vi "radar_plot_tracks.vi"(3 "error in":errorcluster, 5 "Radar Sample":T1) -> (0 "error out":errorcluster)   [LabVIEW 2019, in "Lib_Simx.lvlib"]
doc: "Tool to plot distance away of the radar on the x and y axis."
uses:
  Lib_Simx.lvlib
  controls/radarSample.ctl
  controls/RadarTrack.ctl
  <vilib>/Utility/miscctls.llb/LVAnnotationListTypeDef.ctl
panel:
  in  "Show Track ID":bool
  out "Plot Tracks":cluster{"X1":dbl[], "Y1":dbl[]}[](graph)
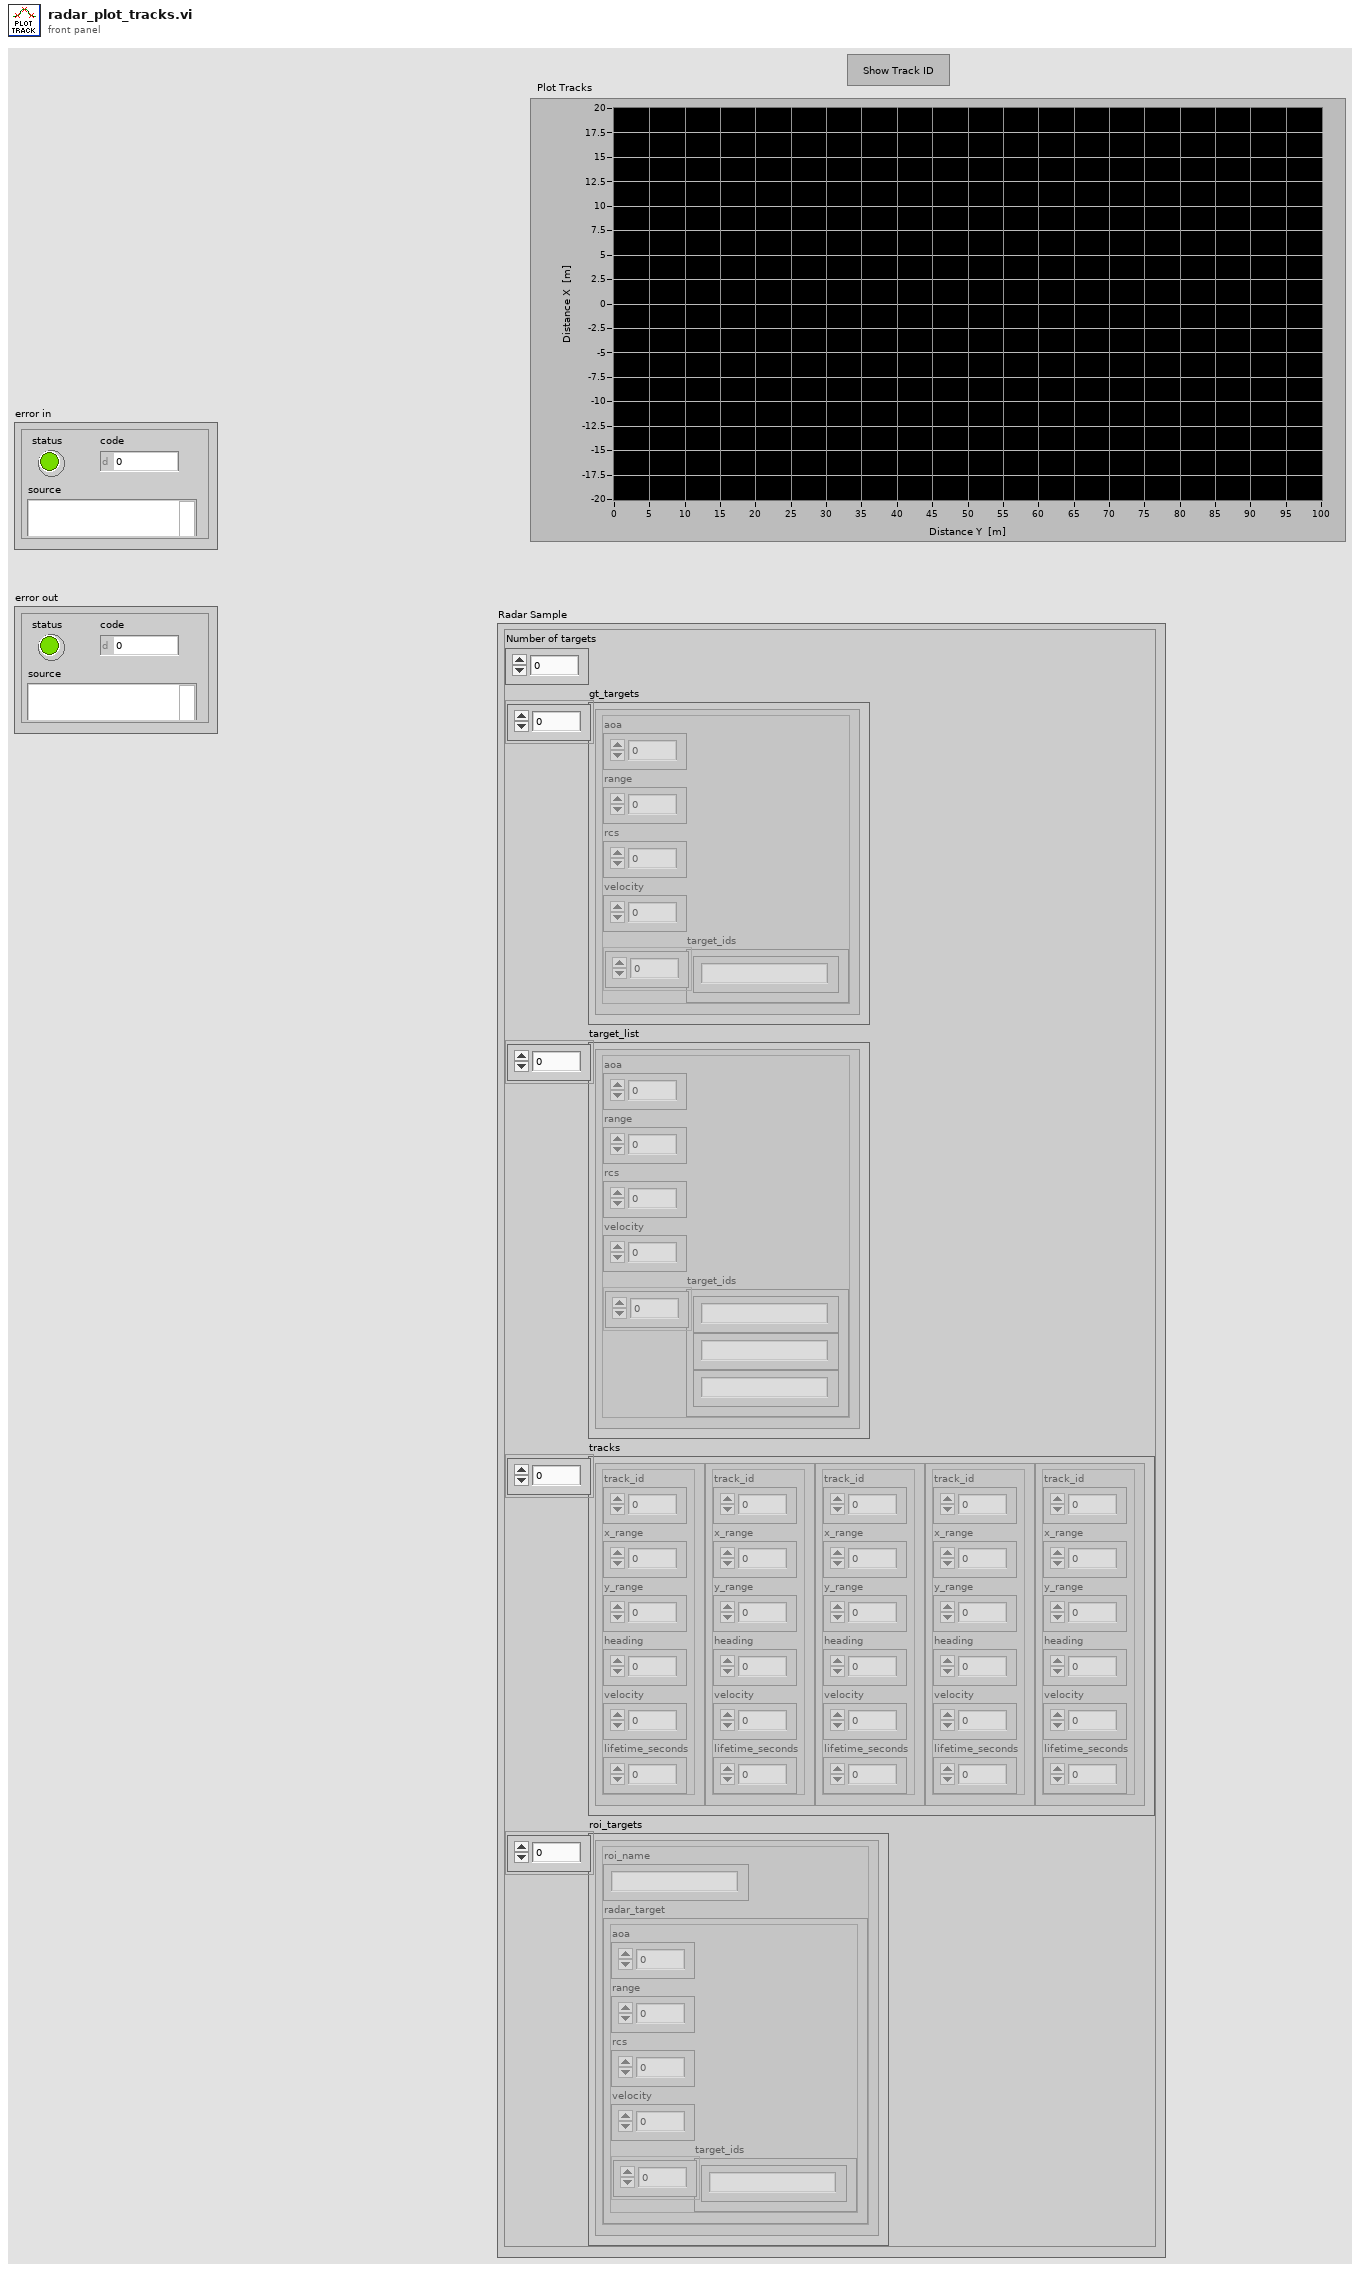
[diagram p1: front panel]
types:
  T1 = typedef "Lib_Simx.lvlib/radarSample.ctl" = cluster{"Number of targets":i32, "gt_targets":cluster{"aoa":sgl, "range":sgl, "rcs":sgl, "velocity":sgl, "target_ids":string[]}[], "target_list":cluster{"aoa":sgl, "range":sgl, "rcs":sgl, "velocity":sgl, "target_ids":string[]}[], "tracks":T2[], "roi_targets":cluster{"roi_name":string, "radar_target":cluster{"aoa":sgl, "range":sgl, "rcs":sgl, "velocity":sgl, "target_ids":string[]}}[]}
  T2 = typedef "Lib_Simx.lvlib/RadarTrack.ctl" = cluster{"track_id":u64, "x_range":sgl, "y_range":sgl, "heading":sgl, "velocity":sgl, "lifetime_seconds":sgl}
  T3 = cluster{"Name":string, "Color":u32, "Style":u8, "Point Style":u8, "Name Visible":bool, "Allow Drag":bool, "Annotation Mode":u32, "Plot":i32, "Index":i32, "Position":cluster{"X":dbl, "Y":dbl}, "X Scale":u32, "Y Scale":u32, "Show Arrow":bool, "Lock Name":bool, "Plot Area":i32, "Label Offset":cluster{"X":dbl, "Y":dbl}}
  T4 = typedef "LVAnnotationListTypeDef.ctl" = cluster{"Name":string, "Color":u32, "Style":u8, "Point Style":u8, "Name Visible":bool, "Allow Drag":bool, "Annotation Mode":u32, "Plot":i32, "Index":i32, "Position":cluster{"X":dbl, "Y":dbl}, "X Scale":u32, "Y Scale":u32, "Show Arrow":bool, "Lock Name":bool, "Plot Area":i32, "Label Offset":cluster{"X":dbl, "Y":dbl}}[]
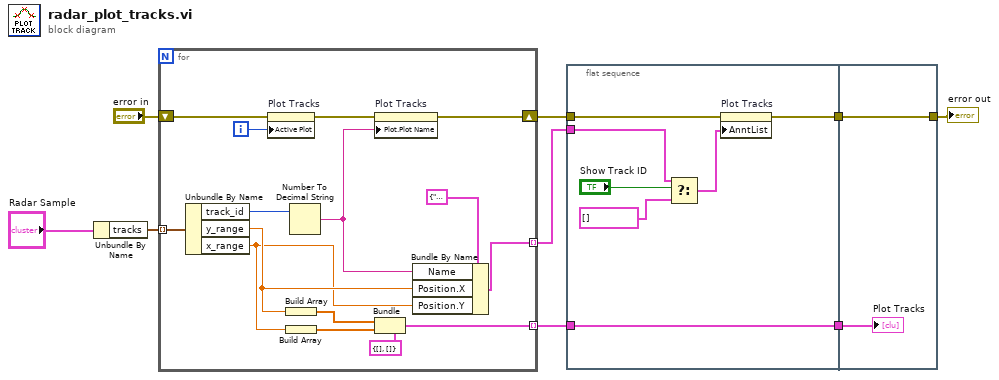
[diagram p0: block diagram]
diagram:
  n1 = Unbundle By Name("Radar Sample") -> ("tracks"=w8:T2[])
  n2 = for {
    tunnel: w8 -> [w24] mode=indexing
    tunnel: [w20] -> w4 mode=indexing
    shift-right: [w10] -> w6
    shift-left: "error in" -> [w17]
    tunnel: [w11] -> w5 mode=indexing
    i -> [w18]
    n3 = Unbundle By Name(w24) -> ("track_id"=w19:u64, "y_range"=w13:sgl, "x_range"=w12:sgl)
    n4 = property on="Plot Tracks" class="XYGraph (strict)"(error in=w17, "Active Plot"=w18) -> (error out=w16:errorcluster)  [unwired: 1 in, 1 out]
    n5 = Build Array(w13) -> (w22:sgl[])
    n6 = Build Array(w12) -> (w21:sgl[])
    n7 = Number To Decimal String(number=w19) -> (decimal integer string=w14:string)  [unwired: 1 in]
    n8 = property on="Plot Tracks" class="XYGraph (strict)"(error in=w16, "Plot.Plot Name"=w14) -> (error out=w10:errorcluster)  [unwired: 1 in, 1 out]
    n9 = Bundle(cluster=cluster{"X1":dbl[], "Y1":dbl[]} {"X1"=[], "Y1"=[]}, "X1"=w22, "Y1"=w21) -> (w20:cluster{"X1":dbl[], "Y1":dbl[]})
    n10 = Bundle By Name(cluster=T3 {"Name"="test", "Color"=16776960, "Style"=4, "Point Style"=13, "Name Visible"=TRUE, "Allow Drag"=TRUE, "Annotation Mode"=0, "Plot"=-1, "Index"=0, "Position"={"X"=65.91230551626592, "Y"=6.291560102301791}, "X Scale"=0, "Y Scale"=0, "Show Arrow"=TRUE, "Lock Name"=FALSE, "Plot Area"=0, "Label Offset"={"X"=0.0, "Y"=2.0460358056265986}}, "Name"=w14, "Position.X"=w13, "Position.Y"=w12) -> (w11:T3)
  }
  n11 = flat-sequence {
    tunnel: w6 -> [w31]
    tunnel: w5 -> [w28]
    tunnel: w4 -> [w30]
    tunnel: [w30] -> w3
    tunnel: [w29] -> w2
    tunnel: w3 -> [w33]
    tunnel: w2 -> [w32]
    tunnel: [w32] -> w1
    frame #0 {
      n12 = Select(t=w28, s="Show Track ID", f=T4 [] ("Annotation List")) -> (s? t:f=w26:T4)
      n13 = property on="Plot Tracks" class="XYGraph (strict)"(error in=w31, "AnntList"=w26) -> (error out=w29:errorcluster)  [unwired: 1 in, 1 out]
    }
    frame #1 {
      "Plot Tracks" <- w33
    }
  }
  "error out" <- w1
